vi "Alarma_VoltToler_IEEE45.vi"(7 "queue_alarmas":refnum<queue>, 11 "Vin":sgl) -> ()   [LabVIEW 2018]
uses:
  Controls/FGV_voltflag_action.ctl
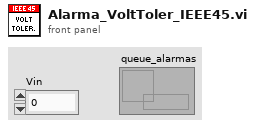
[diagram p1: front panel]
types:
  T1 = typedef "FGV_voltflag_action.ctl" = enum16{"write", "read"}
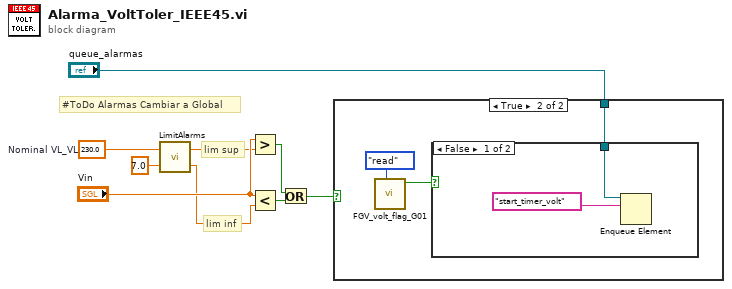
[diagram p0: block diagram]
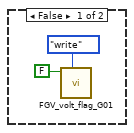
[diagram p2: hidden frame]
diagram:
  w6 = sgl 230.0  # Nominal VL_VL
  # "#ToDo Alarmas Cambiar a Global"
  # "lim inf"
  # "lim sup"
  n1 = call "LimitAlarms.vi"("Value"=sgl 7.0, "Parameter"=w6) -> ("Min"=w8:sgl, "Max"=w7:sgl)
  n2 = Greater?(x="Vin", y=w7) -> (0:w4:bool)
  n3 = Less?(x="Vin", y=w8) -> (x < y?=w5:bool)
  n4 = Or(x=w4, y=w5) -> (x .or. y?=w2:bool)
  n5 = case shown="True" w2 {
    tunnel: "queue_alarmas" -> [_ w12]
    frame False {
      n6 = call "FGV_volt_flag_G01.vi"("Action"=FGV_voltflag_action."write", "flag in"=FALSE) -> ()  [unwired: 8 in, 2 out]
    }
    frame True {
      n7 = call "FGV_volt_flag_G01.vi"("Action"=FGV_voltflag_action."read") -> ("flag out"=w14:bool)  [unwired: 9 in, 1 out]
      n8 = case shown="False" w14 {
        tunnel: w12 -> [w15 _]
        frame False {
          n9 = Enqueue Element(queue=w15, element="start_timer_volt") -> ()  [unwired: 2 in, 3 out]
        }
        frame True {
        }
      }
    }
  }
